vi "Robot Global Data.vi"() -> ()   [LabVIEW 2012]
doc: "This global VI can contain as many global variables as you need. Place a control on the panel, give it a good name. To read or write to it from a VI, drag the icon to the diagram of that VI. You can also drag from the project. Click on the node to change which global you access. You shouldn't have multiple locations writing to a global or it will cause a race-condition."
uses:
  <vilib>/Rock Robotics/WPI/Camera/WPI_CameraImageSize.ctl
  <vilib>/Rock Robotics/WPI/DriverStation/WPI_DriverStationRobotMode2.ctl
panel:
  in  "AngleConst":dbl
  in  "ShooterConst":dbl
  in  "AutoCase":dbl
  in  "BSBotSoftLimit":dbl
  in  "BSTopSoftLimit":dbl
  in  "BallScrewPosition":dbl
  in  "FPyramidVoltConst":dbl
  in  "FPyramidSpeedConst":dbl
  in  "BallScrewCase":i8
  in  "CenterLength":i8
  in  "NewCenter":dbl
  in  "OldThrottle":dbl
  in  "OldDistance":dbl
  in  "BPyramidVoltConst":dbl
  in  "BPyramidSpeedConst":dbl
  in  "Drivetrain Closed\nLoop Max":dbl
  in  "DrivetrainCase":i8
  in  "FVoltConst":dbl
  in  "FSpeedConst":dbl
  in  "BallScrewPID":cluster{"P":dbl, "I":dbl, "D":dbl}
  in  "FrontShooterPID":cluster{"P":dbl, "I":dbl, "D":dbl}
  in  "BackShooterPID":cluster{"P":dbl, "I":dbl, "D":dbl}
  in  "BackRightPID":cluster{"P":dbl, "I":dbl, "D":dbl}
  in  "BackLeftPID":cluster{"P":dbl, "I":dbl, "D":dbl}
  in  "FrontRightPID":cluster{"P":dbl, "I":dbl, "D":dbl}
  in  "FrontLeftPID":cluster{"P":dbl, "I":dbl, "D":dbl}
  in  "ShooterCase":i8
  in  "BackShooterSpeed":dbl
  in  "serial data":string
  in  "Center":dbl=320.0
  in  "Distance":dbl
  in  "Robot Mode":T1
  in  "LED toggle rate (ms)":u32=20
  in  "image size":T2=enum."320x240"
  in  "Enable Vision":bool
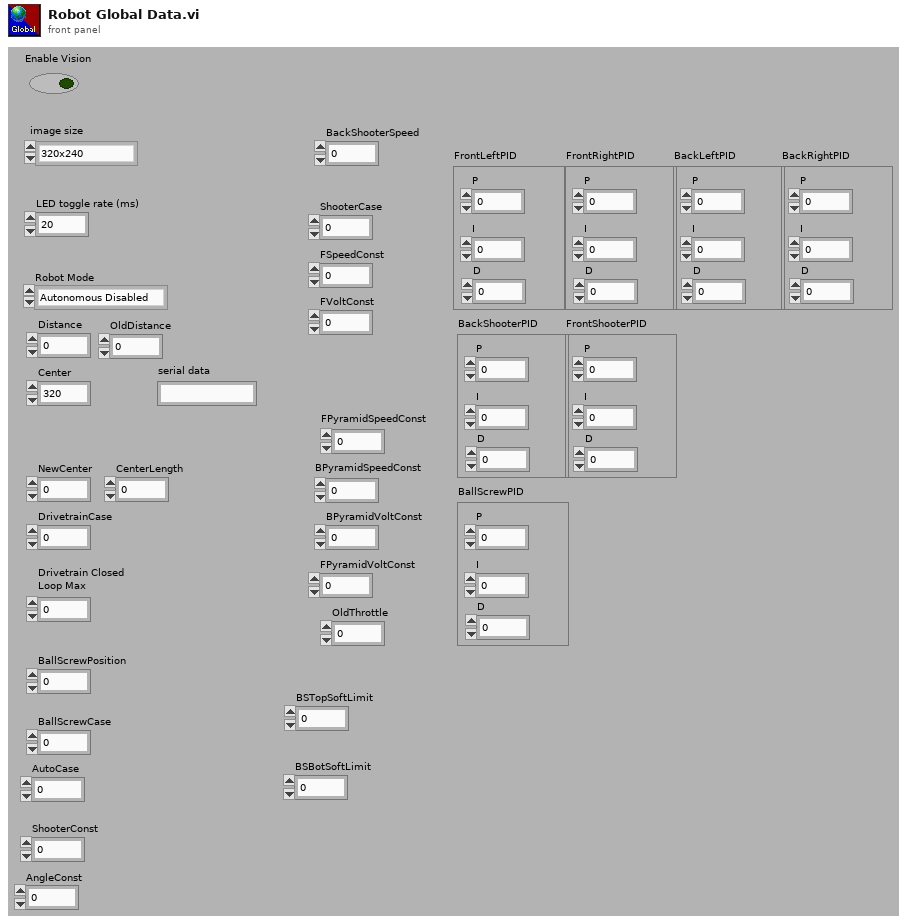
[diagram p1: front panel]
types:
  T1 = typedef "WPI_DriverStationRobotMode2.ctl" = enum16{"Autonomous Disabled", "Autonomous Enabled", "Teleop Disabled", "Teleop Enabled", "Timeout", "Finish", "Test Disabled", "Test Enabled"}
  T2 = typedef "WPI_CameraImageSize.ctl" = enum16{"640x480", "320x240", "160x120"}
diagram:
